vi "Watch Loop Async.vi"(11 "WebProjectWatcher in":refnum<class "WebProjectWatcher.lvclass">) -> ()   [LabVIEW 2020, in "PicoG-Processor.lvlib" / "WebProjectWatcher.lvclass"]
uses:
  WebProjectWatcher.lvclass
  Web Build.ctl
  WebProjectWatcher.lvclass/WebProjectWatcher.ctl
panel:
  out "Builds":T1[](array[typedef]) {"Last Update" format="%<%Y-%m-%d %H:%M:%S>T"}
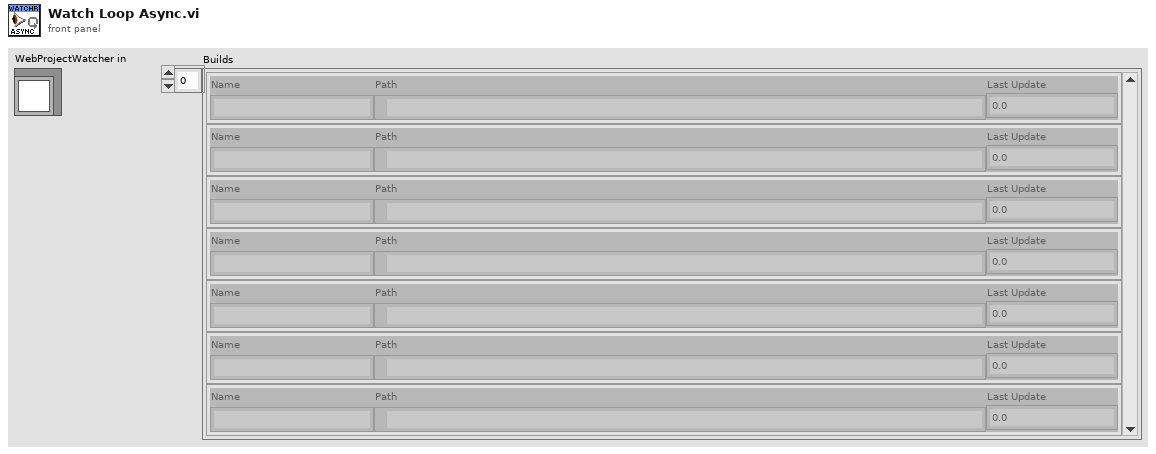
[diagram p1: front panel]
types:
  T1 = typedef "PicoG-Processor.lvlib/WebProjectWatcher.lvclass/Web Build.ctl" = cluster{"Name":string, "Path":path, "Last Update":dbl}
  T2 = typedef "PicoG-Processor.lvlib/WebProjectWatcher.lvclass/Ref Data.ctl" = cluster{"Builds Callbacks":T3[], "Project Path":path, "Close":bool}
  T3 = typedef "PicoG-Processor.lvlib/WebProjectWatcher.lvclass/Builds Callback.ctl" = cluster{"Callback":refnum<vi>, "Owner":refnum<class>}
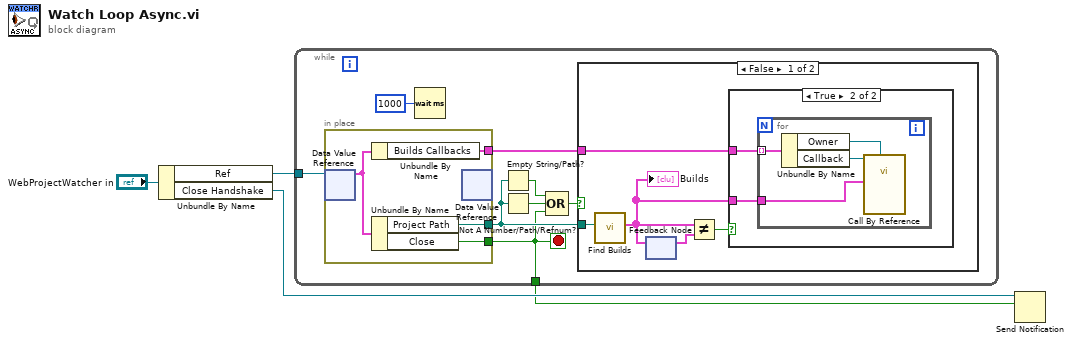
[diagram p0: block diagram]
diagram:
  n1 = Unbundle By Name("WebProjectWatcher in") -> ("Ref"=w3:refnum<data-value>, "Close Handshake"=w2:refnum<notifier>)
  n2 = while {
    tunnel: w3 -> [w6]
    tunnel: [w5] -> w1
    stop <- w5 stop-if-true
    n3 = in-place {
      in-place-border: [w16] -> w8
      in-place-border: [w14] -> w7
      in-place-border: [w13] -> w5
      n4 = in-place-dvr #1(w6) -> (w15:T2)  [unwired: 1 out]
      n5 = Unbundle By Name(w15) -> ("Builds Callbacks"=w14:T3[])
      n6 = Unbundle By Name(w15) -> ("Project Path"=w16:path, "Close"=w13:bool)
      n7 = in-place-dvr #1() -> ()  [unwired: 1 in, 2 out]
    }
    n8 = Wait (ms)(milliseconds to wait=u32 1000) -> ()  [unwired: 1 out]
    n9 = Empty String/Path?(string/path=w8) -> (empty?=w10:bool)
    n10 = Not A Number/Path/Refnum?(number/path/refnum=w8) -> (NaN/Path/Refnum?=w11:bool)
    n11 = Compound Arithmetic op=OR(w10, w11, w5) -> (w9:bool)
    n12 = case shown="False" w9 {
      tunnel: w8 -> [w21 _]
      tunnel: w7 -> [w17 _]
      frame False {
        n13 = call "Find Builds.vi"("Project Path"=w21) -> ("Builds"=w18:T1[])  [unwired: 10 in]
        "Builds" <- w18
        n14 = feedback-in #2(w18) -> ()
        n15 = feedback #2() -> (w20:T1[])  [unwired: 1 in]
        n16 = Not Equal?(x=w18, y=w20) -> (x != y?=w19:bool)
        n17 = case shown="True" w19 {
          tunnel: w18 -> [_ w22]
          tunnel: w17 -> [_ w23]
          frame False {
          }
          frame True {
            n18 = for {
              tunnel: w23 -> [w27] mode=indexing
              tunnel: w22 -> [w24]
              n19 = Unbundle By Name(w27) -> ("Owner"=w25:refnum<class>, "Callback"=w26:refnum<vi>)
              n20 = call-by-ref "?"(reference=w26, "Owner"=w25, "Builds"=w24) -> ()  [unwired: 11 in, 2 out]
            }
          }
        }
      }
      frame True {
      }
    }
  }
  n21 = Send Notification(notification=w1, notifier=w2) -> ()  [unwired: 1 in, 2 out]
